vi "Configure.vi"(8 "error in (no error)":errorcluster) -> (0 "error out":errorcluster, 2 "valid configuration":bool, 3 "config":T1)   [LabVIEW 2017, in "McsaDataEventCreator.lvlib"]
uses:
  <vilib>/addons/InsightCM/Devices/Shared/Mcsa/McsaDataEventCreator/McsaDataEventCreator.lvlib
  <vilib>/addons/InsightCM/Devices/Shared/Mcsa/McsaDataEventCreator/controls/config.ctl
  <vilib>/addons/InsightCM/Devices/Shared/Mcsa/McsaDataEventCreator/controls/DataEventConfig.ctl
  <vilib>/addons/InsightCM/Devices/Shared/Mcsa/McsaDataEventCreator/controls/AcqParams.ctl
  <vilib>/addons/InsightCM/Devices/Shared/Common/DataAccumulator/controls/AccumulationSettings.ctl
  <vilib>/addons/InsightCM/Devices/Shared/Common/DataAccumulator/controls/accumulationType.ctl
  <vilib>/addons/InsightCM/Devices/Shared/Common/DVRBuffer/controls/BufferLocation.ctl
  <vilib>/addons/PointValueMap/controls/PointMap.ctl
  <vilib>/addons/InsightCM/Devices/Shared/Mcsa/McsaDataEventCreator/controls/DataGroupRegistry.ctl
  <vilib>/addons/InsightCM/Devices/Shared/Mcsa/McsaDataEventCreator/controls/Registry_DataSet.ctl
  <vilib>/addons/InsightCM/Devices/Shared/Mcsa/McsaDataEventCreator/controls/DataSetType.ctl
  <vilib>/addons/InsightCM/Devices/Shared/Common/DataEventCreator/controls/Registry_Trend.ctl
  <vilib>/addons/InsightCM/Devices/Shared/Common/DataEvent/controls/Event.ctl
  <vilib>/addons/InsightCM/MessageBus/Base/controls/DataEvent.ctl
  <vilib>/addons/InsightCM/MessageBus/Base/controls/KeyValuePair.ctl
  <vilib>/addons/InsightCM/Devices/Shared/Common/DataEvent/controls/DataSet.ctl
  <vilib>/addons/InsightCM/MessageBus/Base/controls/DataSetMetadata.ctl
  <vilib>/addons/InsightCM/MessageBus/Base/controls/TrendPoint.ctl
  <vilib>/addons/InsightCM/MessageBus/Base/controls/TrendAlarmUpdate.ctl
  <vilib>/addons/InsightCM/MessageBus/Base/controls/TrendAlarmTransition.ctl
  <vilib>/addons/InsightCM/Utilities/GlobalConfiguration/GlobalConfiguration.lvlib
  <vilib>/addons/PointValueMap/PointValueMap.lvlib
  <vilib>/addons/InsightCM/Devices/Shared/Common/DataEventCreator/DataEventCreator.lvlib
  <vilib>/addons/InsightCM/Utilities/PropertyHelpers/PropertyHelpers.lvlib
  <vilib>/addons/InsightCM/Devices/Shared/Common/DVRBuffer/DVRBuffer.lvlib
  <vilib>/addons/InsightCM/Devices/Shared/Common/DataAccumulator/DataAccumulator.lvlib
  <vilib>/addons/InsightCM/Devices/Shared/Mcsa/McsaVirtualChannel/McsaVirtualChannel.lvlib
  <vilib>/addons/InsightCM/Devices/Shared/Common/DataEvent/DataEvent.lvlib
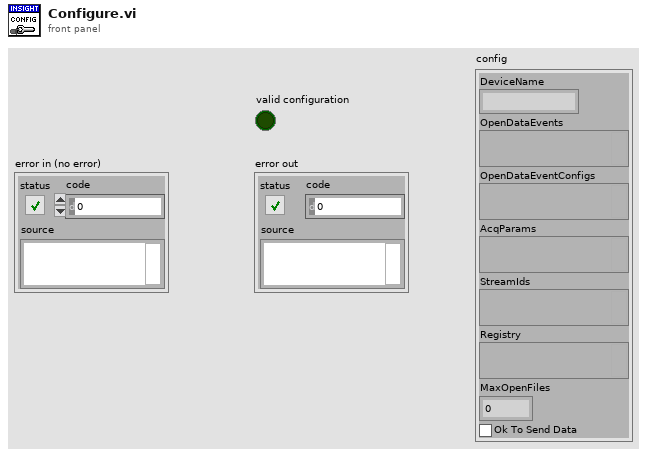
[diagram p1: front panel]
types:
  T1 = typedef "McsaDataEventCreator.lvlib/config.ctl" = cluster{"DeviceName":string, "OpenDataEvents":variant, "OpenDataEventConfigs":variant, "AcqParams":variant, "StreamIds":variant, "Registry":variant, "MaxOpenFiles":i32, "Ok To Send Data":bool}
  T2 = typedef "SectionKeyValues.ctl" = cluster{"Section":string, "KeyValues":T3[]}
  T3 = typedef "KeyValuePair.ctl" = cluster{"Key":string, "Value":string}
  T4 = typedef "R2_Channel.ctl" = cluster{"Id":string, "DeviceId":string, "Name":string, "ChannelType":string, "HardwareKey":string, "HardwareChannel":string, "DataGroup":string, "Keywords":string[], "EquipmentIds":string[], "Properties":T3[], "Metrics":T5[], "AssetNodeId":string, "MeasType":string, "AssetName":string}
  T5 = typedef "Metric.ctl" = cluster{"Id":string, "Name":string, "Unit":string, "Properties":T3[], "MetricDefinitionInstanceId":string}
  T6 = typedef "R2_Device.ctl" = cluster{"Id":string, "Name":string, "DeviceType":string, "HardwareName":string, "IpAddress":string, "HardwareInfo":T3[], "ApplicationType":string, "ApplicationVersion":string, "EquipmentIds":string[], "ConfigurationVersion":string, "State":T7, "Properties":T3[], "DataGroups":T8[], "BurstModeTrigger":T12, "SensorGroups":T13[], "Endpoints":T14[]}
  T7 = typedef "DeviceState.ctl" = cluster{"Disabled":bool}
  T8 = typedef "R2_DataGroup.ctl" = cluster{"Name":string, "OperatingStates":T9[], "Properties":T3[], "EquipmentIds":string[], "AssetNodeId":string}
  T9 = typedef "OperatingState.ctl" = cluster{"Name":string, "Properties":T3[], "Triggers":T10[]}
  T10 = typedef "Trigger.ctl" = cluster{"Type":string, "Expression":string, "Conditions":T11[]}
  T11 = typedef "Condition.ctl" = cluster{"Source":string, "Type":string, "Operator":string, "CompareTo":string, "DwellSeconds":dbl}
  T12 = typedef "BurstModeTrigger.ctl" = cluster{"Trigger":T10, "SampleRate":string, "AcquisitionLength":string}
  T13 = typedef "DeviceSensorGroup.ctl" = cluster{"EquipId":string, "SensorGroupId":string}
  T14 = typedef "WirelessEndpoint.ctl" = cluster{"SerialNumber":string, "Properties":T3[], "Channels":T15[]}
  T15 = typedef "WirelessChannel.ctl" = cluster{"ChannelNumber":i32, "AssetId":string}
  T16 = typedef "DataEvent.lvlib/Event.ctl" = cluster{"DataEvent":T17, "DataSets":T18[], "TrendPoints":T20[], "Alarms":T21[]}
  T17 = typedef "DataEvent.ctl" = cluster{"Id":string, "AssetNodeId":string, "Timestamp":i64, "Props":T3[]}
  T18 = typedef "DataEvent.lvlib/DataSet.ctl" = cluster{"DataSetMetadata":T19, "Values":sgl[], "Values DVR":refnum<data-value>}
  T19 = typedef "DataSetMetadata.ctl" = cluster{"Id":string, "DataEventId":string, "AssetNodeId":string, "Type":string, "T0":i64, "Props":T3[]}
  T20 = typedef "TrendPoint.ctl" = cluster{"TrendPointId":string, "DataEventId":string, "Timestamp":i64, "Value":dbl, "Props":T3[]}
  T21 = typedef "TrendAlarmUpdate.ctl" = cluster{"RuleId":string, "Transition":T22}
  T22 = typedef "TrendAlarmTransition.ctl" = cluster{"At":i64, "Severity":i32, "Value":dbl}
  T23 = typedef "McsaDataEventCreator.lvlib/DataGroupRegistry.ctl" = cluster{"AssetNodeMap":variant, "DataSets":T24[], "Trends":T26[]}
  T24 = typedef "McsaDataEventCreator.lvlib/Registry_DataSet.ctl" = cluster{"ChannelName":string, "DataSetType":T25, "DoNotWriteToDB":bool, "ParentName":string}
  T25 = typedef "McsaDataEventCreator.lvlib/DataSetType.ctl" = enum16{"Waveform", "MCSAFFT", "TorqueWFM"}
  T26 = typedef "DataEventCreator.lvlib/Registry_Trend.ctl" = cluster{"TrendPointId":string, "DataSetName":string, "HighRate":bool, "Always Send":bool}
  T27 = typedef "McsaDataEventCreator.lvlib/DataEventConfig.ctl" = cluster{"AcqParams":T28, "OpState":string, "ExitOpState":bool, "Reason":string, "StreamId":string, "Map":T32, "DataSetIds":variant, "IncludeWaveforms":bool, "TrendPointsOnly":bool}
  T28 = typedef "McsaDataEventCreator.lvlib/AcqParams.ctl" = cluster{"Stream":bool, "PreTrigger":i32, "CollectOnEnter":bool, "Enter PreTrigger":i32, "Enter Length":dbl, "CollectOnExit":bool, "ContinuousData":bool, "Accumulation Settings":T29}
  T29 = typedef "DataAccumulator.lvlib/AccumulationSettings.ctl" = cluster{"Type":T30, "Length":dbl, "Max Time (sec)":dbl, "Start Block":T31, "Acquired (sec)":dbl, "Acquired (pulses)":i32, "Initial Pulse Offset":dbl, "Stop Block":T31, "LastBlockAdded":u32}
  T30 = typedef "DataAccumulator.lvlib/accumulationType.ctl" = enum16{"none", "seconds", "revolutions"}
  T31 = typedef "DVRBuffer.lvlib/BufferLocation.ctl" = cluster{"Block":u32, "Index":i32}
  T32 = typedef "PointValueMap.lvlib/PointMap.ctl" = refnum<data-value>
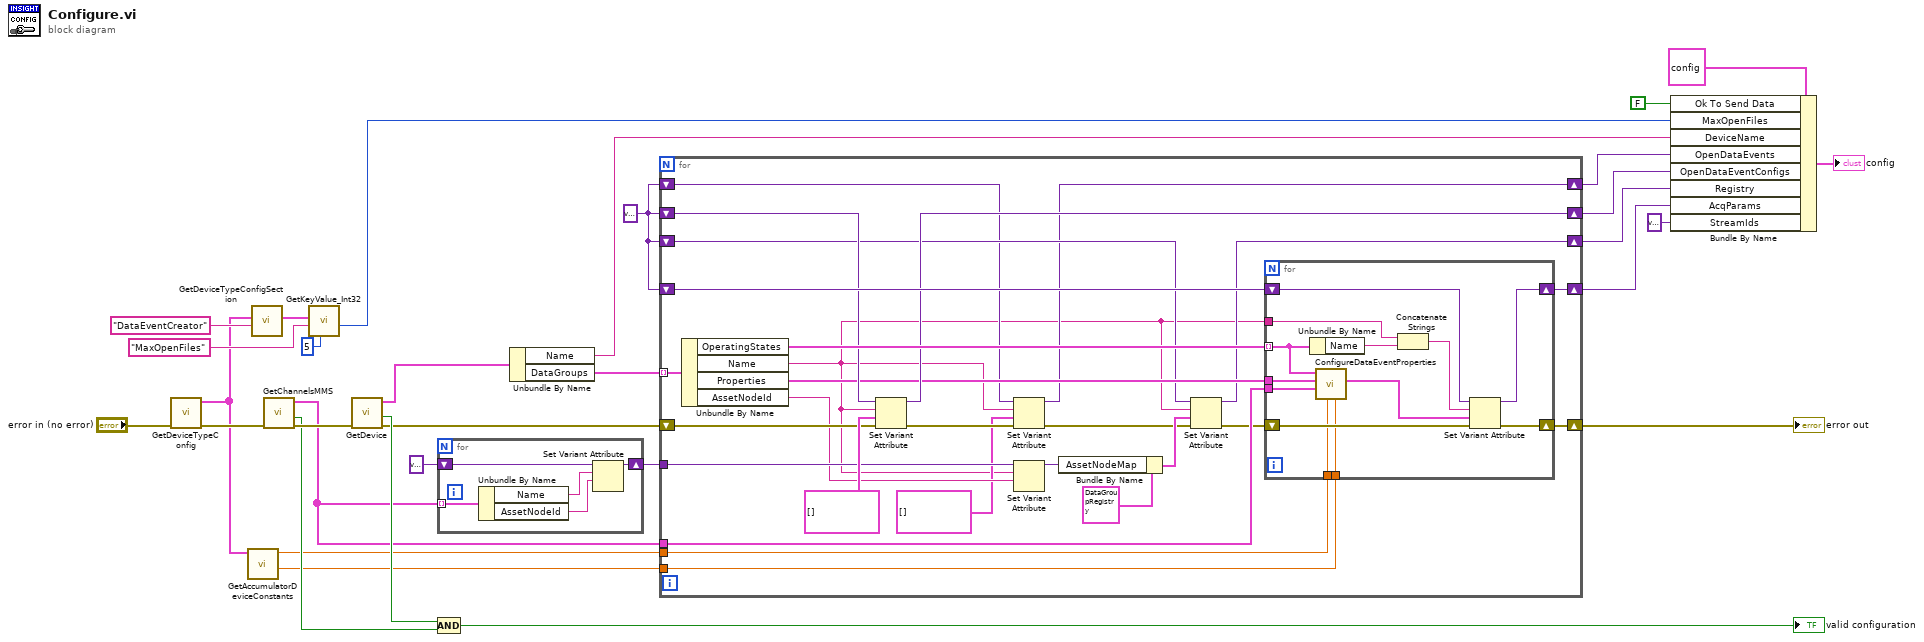
[diagram p0: block diagram]
diagram:
  w3 = variant
  n1 = call <vilib>:"GetDeviceTypeConfig.vi"("error in (no error)"="error in (no error)") -> ("error out"=w15:errorcluster, "key values"=w9:T2[])  [unwired: 8 in, 1 out]
  n2 = call <vilib>:"GetAccumulatorDeviceConstants.vi"("key values"=w9) -> ("default data block length (sec)"=w8:dbl, "max block (sec)"=w6:dbl)  [unwired: 6 in, 3 out]
  n3 = call <vilib>:"GetDeviceTypeConfigSection.vi"("key"="DataEventCreator", "key values"=w9) -> ("key value pairs out"=w13:T3[])  [unwired: 8 in, 1 out]
  n4 = call <vilib>:"GetChannelsMMS.vi"("error in (no error)"=w15) -> ("error out"=w23:errorcluster, "found"=w22:bool, "MMS Channels"=w18:T4[])  [unwired: 6 in, 2 out]
  n5 = call <vilib>:"GetKeyValue_Int32.vi"("default"=5, "key"="MaxOpenFiles", "key value pairs"=w13) -> ("value"=w10:i32)  [unwired: 6 in, 2 out]
  n6 = call <vilib>:"GetDevice.vi"("error in (no error)"=w23) -> ("error out"=w20:errorcluster, "found"=w27:bool, "device configuration"=w30:T6)  [unwired: 8 in]
  n7 = for {
    shift-right: [w34] -> w17
    shift-left: variant -> [w35]
    tunnel: w18 -> [w36] mode=indexing
    n8 = Unbundle By Name(w36) -> ("Name"=w33:string, "AssetNodeId"=w32:string)
    n9 = Set Variant Attribute(Variant=w35, name=w33, value=w32) -> (Variant out=w34:variant)  [unwired: 1 in, 2 out]
  }
  n10 = Compound Arithmetic op=AND(w27, w22) -> (→"valid configuration":bool)
  n11 = Unbundle By Name(w30) -> ("Name"=w24:string, "DataGroups"=w31:T8[])
  n12 = for {
    shift-right: [w52] -> w29
    shift-left: w20 -> [w53]
    tunnel: w31 -> [w62] mode=indexing
    shift-right: [w59] -> w25
    shift-left: w3 -> [w61]
    shift-right: [w57] -> w4
    shift-left: w3 -> [w58]
    tunnel: w18 -> [w54]
    shift-right: [w50] -> w5
    shift-left: w3 -> [w51]
    tunnel: w17 -> [w46]
    tunnel: w8 -> [w44]
    tunnel: w6 -> [w43]
    shift-right: [w38] -> w2
    shift-left: w3 -> [w39]
    n13 = Unbundle By Name(w62) -> ("OperatingStates"=w60:T9[], "Name"=w37:string, "Properties"=w55:T3[], "AssetNodeId"=w45:string)
    n14 = Set Variant Attribute(Variant=w58, name=w37, value=T27[] [], error in=w53) -> (Variant out=w57:variant, error out=w42:errorcluster)  [unwired: 1 out]
    n15 = Set Variant Attribute(Variant=w39, name=w37, value=T16[] [] ("data events"), error in=w42) -> (Variant out=w38:variant, error out=w41:errorcluster)  [unwired: 1 out]
    n16 = Set Variant Attribute(Variant=w46, name=w37, value=w45) -> (Variant out=w47:variant)  [unwired: 1 in, 2 out]
    n17 = Bundle By Name(cluster=T23 {"AssetNodeMap"=variant, "DataSets"=[], "Trends"=[]} ("Data Group Registry"), "AssetNodeMap"=w47) -> (w48:T23)
    n18 = Set Variant Attribute(Variant=w51, name=w37, value=w48, error in=w41) -> (Variant out=w50:variant, error out=w52:errorcluster)  [unwired: 1 out]
    n19 = for {
      shift-right: [w66] -> _
      shift-left: w52 -> [w75]
      shift-right: [w73] -> w59
      shift-left: w61 -> [w74]
      tunnel: w37 -> [w71]
      tunnel: w60 -> [w69] mode=indexing
      tunnel: w55 -> [w68]
      tunnel: w54 -> [w67]
      tunnel: w44 -> [w65]
      tunnel: w43 -> [w64]
      n20 = Unbundle By Name(w69) -> ("Name"=w72:string)
      n21 = call <vilib>:"ConfigureDataEventProperties.vi"("default data block length"=w65, "max time (sec)"=w64, "channels"=w67, "group properties"=w68, "operating state"=w69) -> ("AcqParams"=w63:T28)  [unwired: 6 in]
      n22 = Concatenate Strings(w71, w72) -> (w70:string)
      n23 = Set Variant Attribute(Variant=w74, name=w70, value=w63, error in=w75) -> (Variant out=w73:variant, error out=w66:errorcluster)  [unwired: 1 out]
    }
  }
  "error out" <- w29
  n24 = Bundle By Name(cluster=T1 {"DeviceName"="", "OpenDataEvents"=variant, "OpenDataEventConfigs"=variant, "AcqParams"=variant, "StreamIds"=variant, "Registry"=variant, "MaxOpenFiles"=0, "Ok To Send Data"=FALSE} ("config"), "Ok To Send Data"=FALSE, "MaxOpenFiles"=w10, "DeviceName"=w24, "OpenDataEvents"=w2, "OpenDataEventConfigs"=w4, "Registry"=w5, "AcqParams"=w25, "StreamIds"=variant ("OpStateCorrId")) -> (→"config":T1)
